vi "Array Max & Min (Value).vi"(7 "JSON Value in":refnum<class "JSON Value.lvclass">, 11 "error in (no error)":errorcluster) -> (4 "JSON Value out":refnum<class "JSON Value.lvclass">, 6 "max index":i32, 8 "JSON Value out":refnum<class "JSON Value.lvclass">, 10 "min index":i32, 15 "error out":errorcluster)   [LabVIEW 2016, in "JSON Value.lvclass"]
doc: "Finds the maximum value and minimum value of the elements in a JSON Array. The elements must all be the same literal type."
uses:
  JSON Value.lvclass
  Read Value/Read value (String).vi
  Read Value/Read value (Numeric).vi
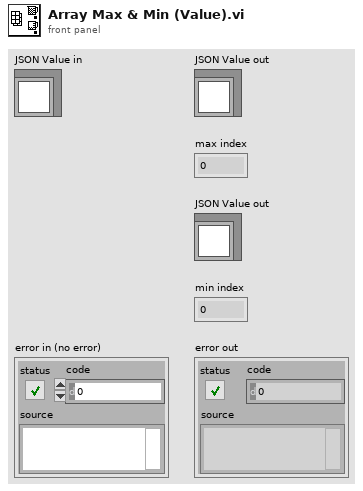
[diagram p1: front panel]
types:
  T1 = typedef "JSON Value.lvclass/JSON Types.ctl" = enum16{"String", "Numeric", "Boolean", "NULL", "Object", "Array"}
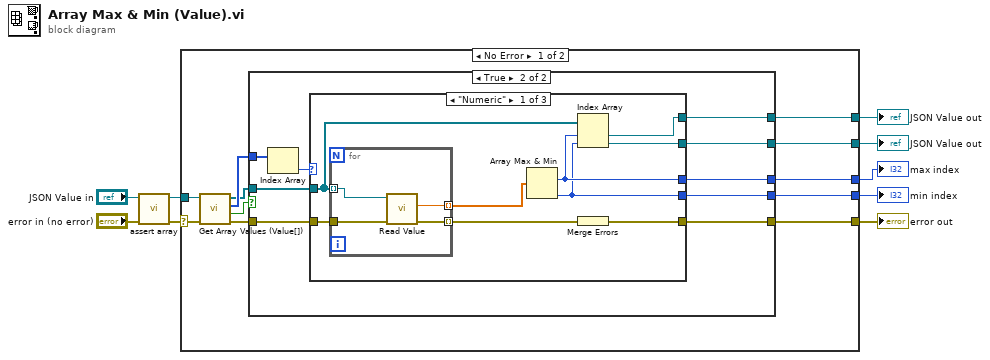
[diagram p0: block diagram]
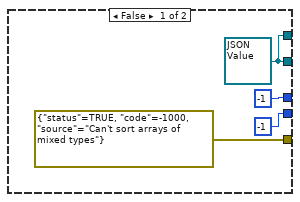
[diagram p2: hidden frame]
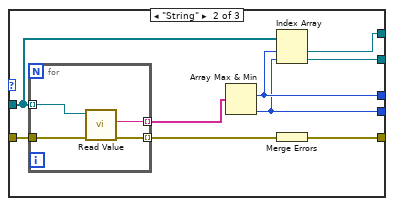
[diagram p3: hidden frame]
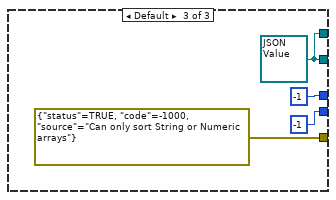
[diagram p4: hidden frame]
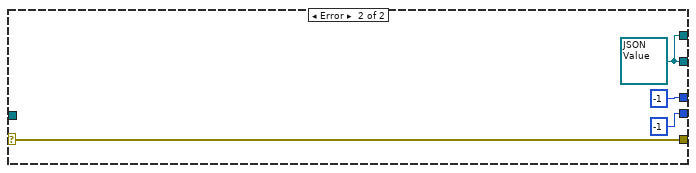
[diagram p5: hidden frame]
diagram:
  n1 = call "assert array.vi"("error in (no error)"="error in (no error)", "JSON Value in"="JSON Value in") -> ("error out"=w3:errorcluster, "JSON Value out"=w1:refnum<class "JSON Value.lvclass">)  [unwired: 8 in]
  n2 = case shown="No Error" w3 {
    selector: w3 -> [w17 w67]
    tunnel: w1 -> [w15 _]
    tunnel: [w20 w67] -> w8
    tunnel: [w13 w64] -> w7
    tunnel: [w12 w64] -> w6
    tunnel: [w11 -1] -> w5
    tunnel: [w10 -1] -> w4
    frame No Error {
      n3 = call "Get Array Values (Value[]).vi"("error in (no error)"=w17, "JSON Value in"=w15) -> ("error out"=w16:errorcluster, "single type?"=w18:bool, "types"=w19:T1[], "values"=w14:refnum<class "JSON Value.lvclass">[])  [unwired: 6 in]
      n4 = case shown="True" w18 {
        tunnel: w14 -> [_ w33]
        tunnel: w16 -> [_ w32]
        tunnel: [errorcluster {"status"=TRUE, "code"=-1000, "source"="Can't sort arrays of mixed types"} ("error IO") w31] -> w20
        tunnel: w19 -> [_ w30]
        tunnel: [w21 w28] -> w13
        tunnel: [w21 w27] -> w12
        tunnel: [-1 w26] -> w11
        tunnel: [-1 w25] -> w10
        frame False {
          w21 = refnum<class "JSON Value.lvclass"> refnum ("JSON Object in")
        }
        frame True {
          n5 = Index Array(array=w30) -> (element=w29:T1)  [unwired: 1 in]
          n6 = case shown="\"Numeric\"" w29 {
            tunnel: w33 -> [w34 w47 _]
            tunnel: w32 -> [w42 w55 _]
            tunnel: [w39 w52 errorcluster {"status"=TRUE, "code"=-1000, "source"="Can only sort String or Numeric arrays"} ("error IO")] -> w31
            tunnel: [w38 w51 w60] -> w28
            tunnel: [w37 w50 w60] -> w27
            tunnel: [w36 w49 -1] -> w26
            tunnel: [w35 w48 -1] -> w25
            frame "Numeric" {
              n7 = for {
                tunnel: w34 -> [w43] mode=indexing
                tunnel: [w46] -> w41 mode=indexing
                tunnel: w42 -> [w45]
                tunnel: [w44] -> w40 mode=indexing
                n8 = call-poly "Read Value.vi"("error in (no error)"=w45, "JSON Numeric in"=w43) -> ("error out"=w44:errorcluster, "value"=w46:dbl)  [unwired: 8 in]
              }
              n9 = Array Max & Min(array=w41) -> (max index (indices)=w36:i32, min index (indices)=w35:i32)  [unwired: 2 out]
              n10 = Index Array(array=w34, index #1=w36, index #2=w35) -> (element #1=w38:refnum<class "JSON Value.lvclass">, element #2=w37:refnum<class "JSON Value.lvclass">)
              n11 = Merge Errors(w40) -> (w39:errorcluster)
            }
            frame "String" {
              n12 = for {
                tunnel: w47 -> [w56] mode=indexing
                tunnel: [w59] -> w54 mode=indexing
                tunnel: w55 -> [w58]
                tunnel: [w57] -> w53 mode=indexing
                n13 = call-poly "Read Value.vi"("error in (no error)"=w58, "JSON String in"=w56) -> ("error out"=w57:errorcluster, "value"=w59:string)  [unwired: 8 in]
              }
              n14 = Array Max & Min(array=w54) -> (max index (indices)=w49:i32, min index (indices)=w48:i32)  [unwired: 2 out]
              n15 = Index Array(array=w47, index #1=w49, index #2=w48) -> (element #1=w51:refnum<class "JSON Value.lvclass">, element #2=w50:refnum<class "JSON Value.lvclass">)
              n16 = Merge Errors(w53) -> (w52:errorcluster)
            }
            frame Default {
              w60 = refnum<class "JSON Value.lvclass"> refnum ("JSON Object in")
            }
          }
        }
      }
    }
    frame Error {
      w64 = refnum<class "JSON Value.lvclass"> refnum ("JSON Object in")
    }
  }
  "error out" <- w8
  "JSON Value out" <- w7
  "JSON Value out" <- w6
  "max index" <- w5
  "min index" <- w4
